vi "PH_SRDG645.evt Call Set Output.vi"(0 "i ref in":refnum<vi>, 1 "Generator Instance":string="N/A", 2 "Output BNC":T1 items=["T0", "AB", "CD", "EF", "GH"], 3 "Output Settings":T2={"Level Offset [V]"=0.0, "Amplitue [V]"=1000.0, "Polarity"=1} {"Polarity" items=["negative", "positive"]}, 5 "error IO":errorcluster) -> (14 "i ref out":refnum<vi>, 19 "error out":errorcluster)   [LabVIEW 2014, in "PH_SRDG645.lvlib"]
doc: "This VI sends a simple event call."
uses:
  PH_SRDG645.lvlib
  instr.lib/Stanford Research DG645/Driver/Output BNC.ctl
  CSCore/CSSystem/CoreLib/CoreLib.int 2 byte array.vi
  CSCore/CSSystem/CoreLib/CoreLib.double 2 byte array.vi
  CSCore/CSSystem/CoreLib/CoreLib.lvlib
  CSCore/BaseProcess/BaseProcess.lvlib
  instr.lib/Stanford Research DG645/Stanford Research DG645 - Driver.lvlib
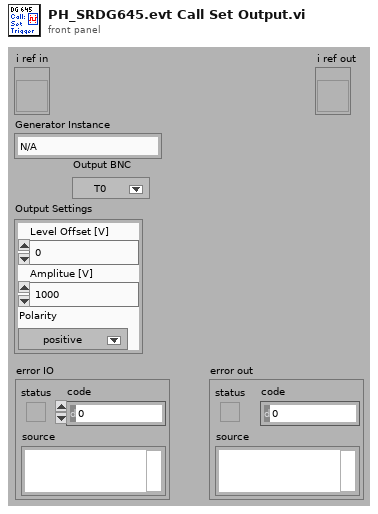
[diagram p1: front panel]
types:
  T1 = typedef "Stanford Research DG645 - Driver.lvlib/Output BNC.ctl" = i32
  T2 = cluster{"Level Offset [V]":dbl, "Amplitue [V]":dbl, "Polarity":i32}
  T3 = typedef "CoreDefs.rawDataType.ctl" = i8[]
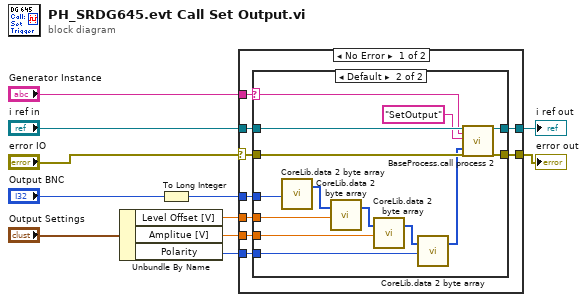
[diagram p0: block diagram]
diagram:
  n1 = Unbundle By Name("Output Settings") -> ("Level Offset [V]"=w5:dbl, "Amplitue [V]"=w4:dbl, "Polarity"=w3:i32)
  n2 = To Long Integer(number="Output BNC") -> (32bit integer=w1:T1)
  n3 = case shown="No Error" "error IO" {
    selector: "error IO" -> [w20 w37]
    tunnel: "Generator Instance" -> [w13 _]
    tunnel: [w19 w37] -> w11
    tunnel: [w17 w38] -> w10
    tunnel: w3 -> [w14 _]
    tunnel: w4 -> [w15 _]
    tunnel: w5 -> [w16 _]
    tunnel: "i ref in" -> [w18 w38]
    tunnel: w1 -> [w12 _]
    frame No Error {
      n4 = case shown="Default" w13 {
        selector: w13 -> [_ w29]
        tunnel: w20 -> [w21 w36]
        tunnel: [w21 w35] -> w19
        tunnel: w18 -> [w22 w34]
        tunnel: [w22 w33] -> w17
        tunnel: w16 -> [_ w26]
        tunnel: w15 -> [_ w28]
        tunnel: w14 -> [_ w27]
        tunnel: w12 -> [_ w23]
        frame "", "N/A" {
        }
        frame Default {
          n5 = call-poly "CoreLib.data 2 byte array.vi"("i32"=w23) -> ("byteArray out"=w24:T3)  [unwired: 18 in]
          n6 = call-poly "CoreLib.data 2 byte array.vi"("byteArray"=w24, "f64"=w26) -> ("byteArray out"=w31:T3)  [unwired: 17 in]
          n7 = call-poly "CoreLib.data 2 byte array.vi"("byteArray"=w31, "f64"=w28) -> ("byteArray out"=w30:T3)  [unwired: 17 in]
          n8 = call-poly "CoreLib.data 2 byte array.vi"("byteArray"=w30, "i32"=w27) -> ("byteArray out"=w25:T3)  [unwired: 17 in]
          n9 = call "BaseProcess.call process 2.vi"("i ref in"=w34, "Object"=w29, "Selector"="SetOutput", "Data"=w25, "error in (no error)"=w36) -> ("i ref out"=w33:refnum<vi>, "error out"=w35:errorcluster)  [unwired: 13 in]
        }
      }
    }
    frame Error {
    }
  }
  "error out" <- w11
  "i ref out" <- w10
